vi "DSF.Engine.Buffer Converter.Get Channels Buffer.vi"(11 "Buffer Converter in":refnum<class "Buffer Converter.lvclass">) -> (2 "channels buffer":dbl[](array[numeric]), 3 "Buffer Converter out":refnum<class "Buffer Converter.lvclass">)   [LabVIEW 2017, in "DSF.Engine.lvlib" / "Buffer Converter.lvclass"]
uses:
  Buffer Converter.lvclass
  Buffer Converter.lvclass/Buffer Converter.ctl
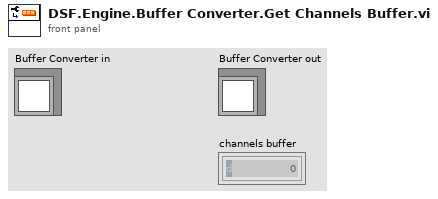
[diagram p1: front panel]
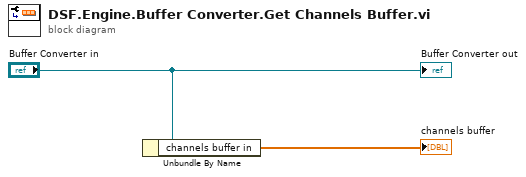
[diagram p0: block diagram]
diagram:
  n1 = Unbundle By Name("Buffer Converter in") -> ("channels buffer in"=→"channels buffer":dbl[])
  "Buffer Converter out" <- "Buffer Converter in"
